vi "TimeDate to URL With Airport.vi"(10 "Time Stamp":timestamp, 11 "Airport Code":string) -> (3 "URL":string)   [LabVIEW 2012]
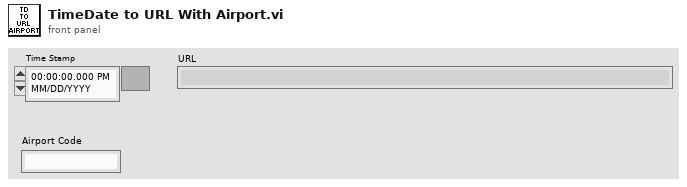
[diagram p1: front panel]
types:
  T1 = typedef "LVDateTimeRec.ctl" = cluster{"fractional second":dbl, "second":i32, "minute":i32, "hour":i32, "day of month":i32, "month":i32, "year":i32, "day of week":i32, "day of year":i32, "DST":i32}
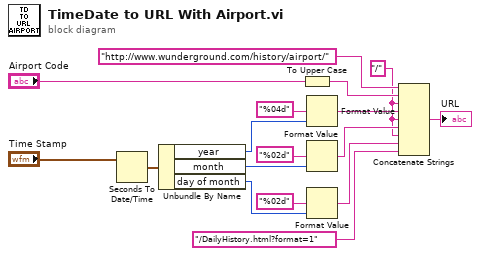
[diagram p0: block diagram]
diagram:
  w4 = "/" ("string")
  n1 = Seconds To Date/Time(time stamp (now)="Time Stamp") -> (date time rec=w16:T1)  [unwired: 1 in]
  n2 = Unbundle By Name(w16) -> ("year"=w15:i32, "month"=w11:i32, "day of month"=w10:i32)
  n3 = To Upper Case(1:"Airport Code") -> (0:w8:string)
  n4 = Format Value(format string="%04d", value (0)=w15) -> (output string=w6:string)  [unwired: 1 in]
  n5 = Format Value(format string="%02d", value (0)=w11) -> (output string=w5:string)  [unwired: 1 in]
  n6 = Format Value(format string="%02d", value (0)=w10) -> (output string=w3:string)  [unwired: 1 in]
  n7 = Concatenate Strings("http://www.wunderground.com/history/airport/", w8, w4, w6, w4, w5, w4, w3, "/DailyHistory.html?format=1") -> (→"URL":string)
